vi "Set Master.vi"(0 "Register Buses":refnum<class "ni579x Register Bus v1 Host.lvclass">[](array[class]), 11 "error in":errorcluster) -> (4 "Register Buses (out)":refnum<class "ni579x Register Bus v1 Host.lvclass">[](array[class]), 15 "error out":errorcluster)   [LabVIEW 2012, in "ni579x Synchronization v1 Host.lvlib"]
doc: "Set the first FPGA in the array of FPGA VI References as the synchronization master."
uses:
  <instrlib>/ni579x/Synchronization/v1/Host/ni579x Synchronization v1 Host.lvlib
  <instrlib>/ni579x/Register Bus/v1/Host/ni579x Register Bus v1 Host.lvclass
  <instrlib>/ni579x/Synchronization/v1/Shared/ni579x Synchronization Register Addresses.ctl
  <instrlib>/ni579x/Register Bus/v1/Host/Public/Register Write.ctl
  <instrlib>/ni579x/Config/v1/Shared/Types/ni579x Register Bus Subsystem ID.ctl
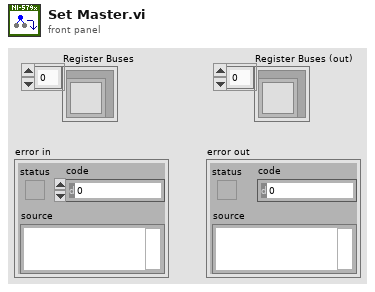
[diagram p1: front panel]
types:
  T1 = typedef "ni579x Register Bus v1 Host.lvclass/Register Write.ctl" = cluster{"subsystem":u8, "address":u16, "data":u32}
  T2 = typedef "ni579x Synchronization Register Addresses.ctl" = enum16{"Signature", "Current Version", "Oldest Compatible Version", "Scratch Register", "sync.master", "sync.meas.enable", "sync.meas.ready", "sync.meas.arm", "sync.meas.valid", "sync.meas.value", "sync.cptr.adjust", "sync.cptr.period", "sync.meas.oversample factor"}
  T3 = typedef "ni579x Register Bus Subsystem ID.ctl" = u8
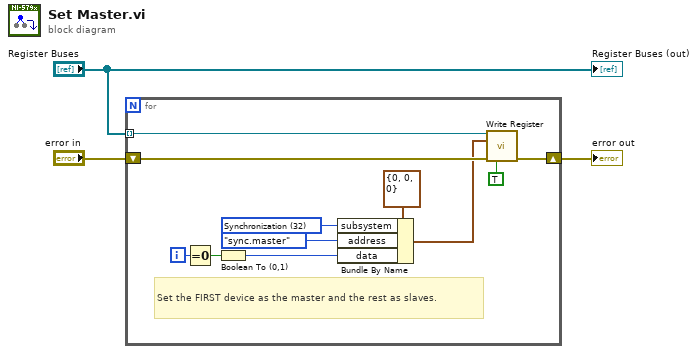
[diagram p0: block diagram]
diagram:
  n1 = for {
    tunnel: "Register Buses" -> [w14] mode=indexing
    shift-right: [w11] -> w1
    shift-left: "error in" -> [w13]
    i -> [w5]
    w8 = T3 32 items=["FAM Register Operation"=0, "User Command"=16, "Synchronization"=32] ("Subsystem ID")
    # "Set the FIRST device as the master and the rest as slaves."
    n2 = Equal To 0?(x=w5) -> (x = 0?=w6:bool)
    n3 = Boolean To (0,1)(Boolean=w6) -> (0, 1=w10:i16)
    n4 = Bundle By Name(cluster=T1 {"subsystem"=0, "address"=0, "data"=0} ("register write"), "subsystem"=w8, "address"=ni579x_Synchronization_Register_Addresses."sync.master" ("Synchronization Registers"), "data"=w10) -> (w4:T1)
    n5 = call <instrlib>:"Write Register.vi"("session in"=w14, "register write"=w4, "error in"=w13, "wait until committed"=TRUE) -> ("error out"=w11:errorcluster)  [unwired: 10 in, 1 out]
  }
  "error out" <- w1
  "Register Buses (out)" <- "Register Buses"
